vi "PH_Tektronix_7000.Set Channel Name BG Color.vi"(0 "i ref in":refnum<vi>, 5 "error in":errorcluster) -> (14 "i ref out":refnum<vi>, 19 "error out":errorcluster)   [LabVIEW 2014, in "PH_Tektronix_7000.lvlib"]
doc: "This VI sets the background color of the channel name to fit to the color correspond to color chosen at the graph."
uses:
  PH_Tektronix_7000.lvlib
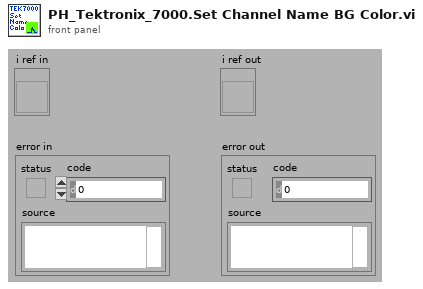
[diagram p1: front panel]
types:
  T1 = typedef "PH_Tektronix_7000.lvlib/PH_Tektronix_7000.i attribute.ctl" = cluster{"VISA Resource Name":refnum<visa-resource-name>, "IDN":cluster{"Instrument Driver":string, "Instrument Firmware":string, "Model":string, "Serial Number":string}, "Selftest":cluster{"Result":i32, "Message":string}, "Trigger Configuration":T2, "Acquisition Configuration":T3, "GUI Refs":T4, "State":T5, "Error Message":string, "Allow Prdc Loop?":bool, "Channel 1":T6, "Channel 2":T6, "Channel 3":T6, "Channel 4":T6, "Data CH 1":waveform(dbl), "Data CH 2":waveform(dbl), "Data CH 3":waveform(dbl), "Data CH 4":waveform(dbl), "Allow config?":bool, "Name Channel 1":string, "Name Channel 2":string, "Name Channel 3":string, "Name Channel 4":string, "Fetch Data before sending to PSDB?":bool, "Constructor passed?":bool, "Data taken at":timestamp, "Plot Colors":u32[], "Default VISA Resource":string}
  T2 = typedef "PH_Tektronix_7000.lvlib/PH_Tektronix_7000.Trigger Config.ctl" = cluster{"Source":u16, "Level [V]":dbl, "Slope":u16, "Coupling":u16, "Trigger Mode":u16}
  T3 = typedef "PH_Tektronix_7000.lvlib/PH_Tektronix_7000.Acquisition Config.ctl" = cluster{"Record Length":u32, "Timebase [s/div]":dbl, "Position [%]":dbl, "Acquisition Type":u16, "Average Waveforms":i32, "Envelope Waveforms":i32, "WfmDB Samples":i32, "Continuous?":bool, "Delay [s]":dbl, "Run?":bool}
  T4 = typedef "PH_Tektronix_7000.lvlib/PH_Tektronix_7000.GUI Refs.ctl" = cluster{"Graph":refnum<vi>, "State":refnum<vi>, "Delete":refnum<vi>, "VISA Resource":refnum<vi>, "Allow Configure":refnum<vi>, "Fetch Data":refnum<vi>, "Fetch before sending Data to PSDB":refnum<vi>, "Name Channel 1":refnum<vi>, "Name Channel 2":refnum<vi>, "Name Channel 3":refnum<vi>, "Name Channel 4":refnum<vi>, "Prdc Intervall [ms]":refnum<vi>, "Data taken":refnum<vi>, "Model":refnum<vi>, "Serial Number":refnum<vi>, "Firmware":refnum<vi>, "Driver":refnum<vi>, "Acquisition":refnum<vi>, "Trigger":refnum<vi>, "Cursor: D Time [s]":refnum<vi>, "Cursor: D Signal [V]":refnum<vi>, "Channel 1":refnum<vi>, "Channel 2":refnum<vi>, "Channel 3":refnum<vi>, "Channel 4":refnum<vi>}
  T5 = typedef "PH_StatusHandler.lvlib/PH_StatusHandler.Status.ctl" = i16
  T6 = typedef "PH_Tektronix_7000.lvlib/PH_Tektronix_7000.Channel Config.ctl" = cluster{"Enable Channel":bool, "Bandwidth":u16, "Input Impedance":u16, "Vertical Coupling":u16, "Probe Attenuation":dbl, "Range [V/div]":dbl, "Position [div]":dbl, "Bandwidth raw":string}
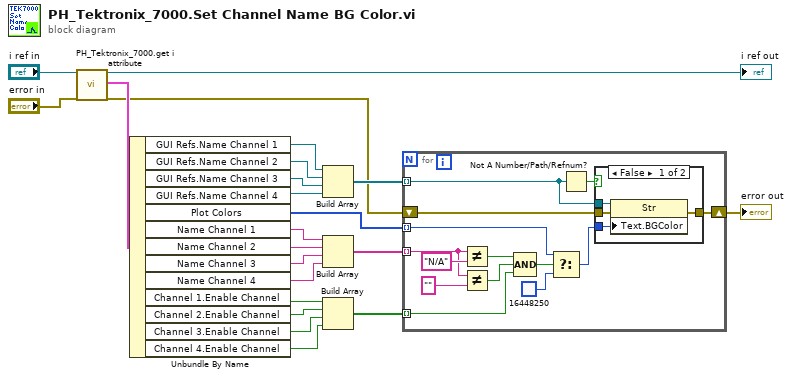
[diagram p0: block diagram]
diagram:
  n1 = call "PH_Tektronix_7000.get i attribute.vi"("i ref in"="i ref in", "error in (no error)"="error in") -> ("i ref out"=→"i ref out":refnum<vi>, "i attribute"=w18:T1, "error out"=w12:errorcluster)  [unwired: 15 in]
  n2 = Unbundle By Name(w18) -> ("GUI Refs.Name Channel 1"=w17:refnum<vi>, "GUI Refs.Name Channel 2"=w16:refnum<vi>, "GUI Refs.Name Channel 3"=w15:refnum<vi>, "GUI Refs.Name Channel 4"=w14:refnum<vi>, "Plot Colors"=w1:u32[], "Name Channel 1"=w9:string, "Name Channel 2"=w8:string, "Name Channel 3"=w7:string, "Name Channel 4"=w10:string, "Channel 1.Enable Channel"=w6:bool, "Channel 2.Enable Channel"=w5:bool, "Channel 3.Enable Channel"=w4:bool, "Channel 4.Enable Channel"=w11:bool)
  n3 = Build Array(w17, w16, w15, w14) -> (w13:refnum<vi>[])
  n4 = Build Array(w9, w8, w7, w10) -> (w3:string[])
  n5 = Build Array(w6, w5, w4, w11) -> (w2:bool[])
  n6 = for {
    shift-right: [w36] -> w19
    shift-left: w12 -> [w35]
    tunnel: w13 -> [w33] mode=indexing
    tunnel: w3 -> [w31] mode=indexing
    tunnel: w2 -> [w27] mode=indexing
    tunnel: w1 -> [w24] mode=indexing
    n7 = Not Equal?(x=w31, y="N/A") -> (x != y?=w29:bool)
    n8 = Not Equal?(x=w31, y="") -> (x != y?=w28:bool)
    n9 = Compound Arithmetic op=AND(w29, w28, w27) -> (w26:bool)
    n10 = Select(t=w24, s=w26, f=u32 16448250 ("Color Box")) -> (s? t:f=w23:u32)
    n11 = Not A Number/Path/Refnum?(number/path/refnum=w33) -> (NaN/Path/Refnum?=w34:bool)
    n12 = case shown="False" w34 {
      tunnel: [w40 w41] -> w36
      tunnel: w35 -> [w39 w41]
      tunnel: w33 -> [w38 _]
      tunnel: w23 -> [w37 _]
      frame False {
        n13 = property class="Str"(reference=w38, error in=w39, "Text.BGColor"=w37) -> (error out=w40:errorcluster)  [unwired: 1 out]
      }
      frame True {
      }
    }
  }
  "error out" <- w19
